vi "Semitransparent PNG Overlay.vi"(7 "Transparency Factor":sgl(slide)=0.5 scale=0.0..1.0, 8 "Overlay Image":path) -> (3 "Image":T1(plugin-control))   [LabVIEW 2012]
doc: "The Grab VI acquires images continuously and displays the images in an image control using low-level acquisition VIs. A grab is appropriate for high-speed applications in which you need to process only one image at a time."
panel:
  in  "Background Image":path
  in  "Coordinates of Overlay":cluster{"x-coord":i32, "y-coord":i32}={"x-coord"=100, "y-coord"=100}
  in  "stop":bool
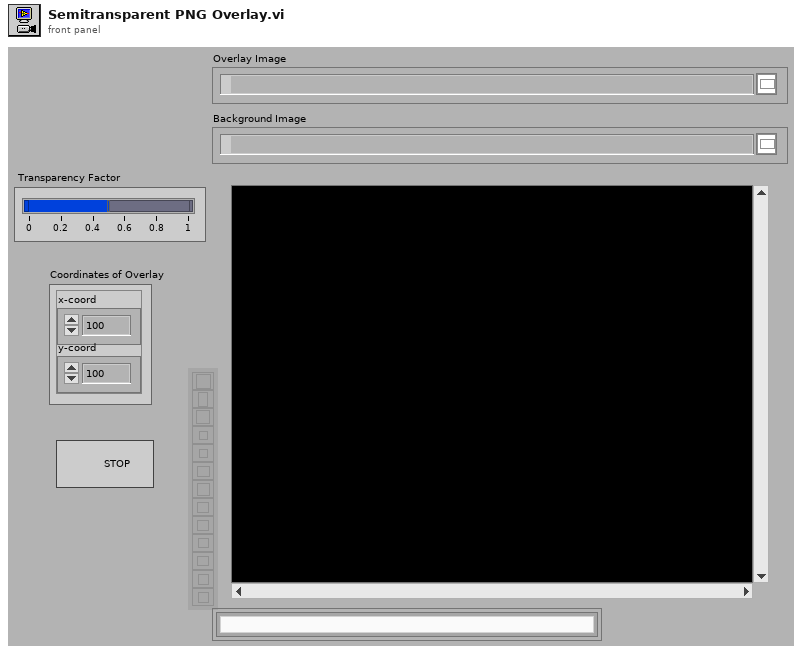
[diagram p1: front panel]
types:
  T1 = typedef "IMAQ Image.ctl" = refnum<image>
  T2 = typedef "Image Type" = u32
  T3 = typedef "imagedata.ctl" = cluster{"image type":i32, "image depth":i32, "image":u8[], "mask":u8[], "colors":u32[], "Rectangle":cluster{"left":i16, "top":i16, "right":i16, "bottom":i16}}
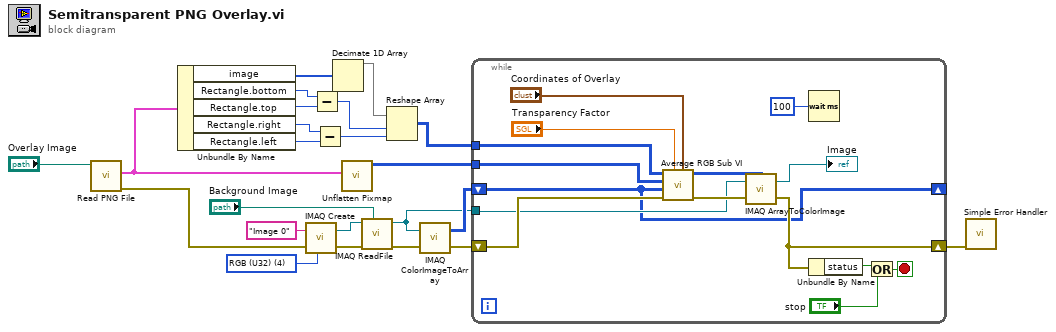
[diagram p0: block diagram]
diagram:
  w5 = T2 4 items=["Grayscale (U8)", "Grayscale (I16)", "Grayscale (SGL)", "Complex (CSG)", "RGB (U32)", "HSL (U32)", "RGB (U64)", "Grayscale (U16)"] ("Image Type")
  n1 = call <vilib>:"Read PNG File.vi"("path to PNG file"="Overlay Image") -> ("error out"=w8:errorcluster, "image data"=w21:T3)  [unwired: 8 in, 1 out]
  n2 = Unbundle By Name(w21) -> ("image"=w20:u8[], "Rectangle.bottom"=w19:i16, "Rectangle.top"=w18:i16, "Rectangle.right"=w12:i16, "Rectangle.left"=w15:i16)
  n3 = call "IMAQ Create"("Image Name"="Image 0", "Image Type"=w5, "error in (no error)"=w8) -> ("New Image"=w10:T1, "error out"=w9:errorcluster)  [unwired: 1 in, 1 out]
  n4 = Subtract(x=w19, y=w18) -> (x-y=w16:i16)
  n5 = Subtract(x=w12, y=w15) -> (x-y=w14:i16)
  n6 = Decimate 1D Array(w20) -> (w17:u8[])  [unwired: 3 out]
  n7 = call <vilib>:"Unflatten Pixmap.vi"("image data"=w21) -> ("24-bit pixmap"=w22:u32[][])  [unwired: 4 in, 6 out]
  n8 = call "IMAQ ReadFile"("File Path"="Background Image", "error in (no error)"=w9, "Image"=w10) -> ("error out"=w4:errorcluster, "Image Out"=w1:T1)  [unwired: 4 in, 3 out]
  n9 = Reshape Array(w17, w16, w14) -> (w13:u8[][])
  n10 = call "IMAQ ColorImageToArray"("Image"=w1, "error in (no error)"=w4) -> ("Image Pixels (U32)"=w2:u32[][], "error out"=w3:errorcluster)  [unwired: 2 in, 1 out]
  n11 = while {
    tunnel: w22 -> [w33]
    shift-right: [w28] -> w11
    shift-left: w3 -> [w27]
    tunnel: w13 -> [w32]
    shift-right: [w25] -> _
    shift-left: w2 -> [w25]
    tunnel: w1 -> [w26]
    stop <- w38 stop-if-true
    n12 = call "Average RGB Sub VI.vi"("Coordinates of Overlay"="Coordinates of Overlay", "Transparency Factor"="Transparency Factor", "error in"=w27, "Image"=w25, "Overlay"=w33, "Alpha Values (Transparency)"=w32) -> ("error out"=w34:errorcluster, "Image Out"=w35:u32[][])  [unwired: 4 in]
    n13 = call "IMAQ ArrayToColorImage"("Image Pixels (U32)"=w35, "Image"=w26, "error in (no error)"=w34) -> ("Image Out"=→"Image":T1, "error out"=w28:errorcluster)  [unwired: 2 in]
    n14 = Wait (ms)(milliseconds to wait=u32 100) -> ()  [unwired: 1 out]
    n15 = Unbundle By Name(w28) -> ("status"=w37:bool)
    n16 = Or(x=w37, y="stop") -> (x .or. y?=w38:bool)
  }
  n17 = call <vilib>:"Simple Error Handler.vi"("error in (no error)"=w11) -> ()  [unwired: 4 in, 5 out]
